vi "grab image.vi"(8 "error in (no error)":errorcluster, 10 "Image In":T1, 11 "Camera":T2) -> (0 "error out":errorcluster, 2 "Image Out":T1, 3 "Camera out":T2)   [LabVIEW 2022 SP3, in "Vision.lvlib"]
uses:
  Vision.lvlib
  camera.ctl
  camera driver.ctl
  <vilib>/vision/Image Controls.llb/IMAQ Image.ctl
  <vilib>/userDefined/High Color/IMAQdx.ctl
  C:/Users/Caleb/Desktop/nebraska-silicon-lab/pixel-gantry-control/Gantry/Shared Components/bin/uEyeDotNet.dll
  bin/uEyeDotNet.dll
  <vilib>/vision/driver/NI_Vision_Acquisition_Software.lvlib
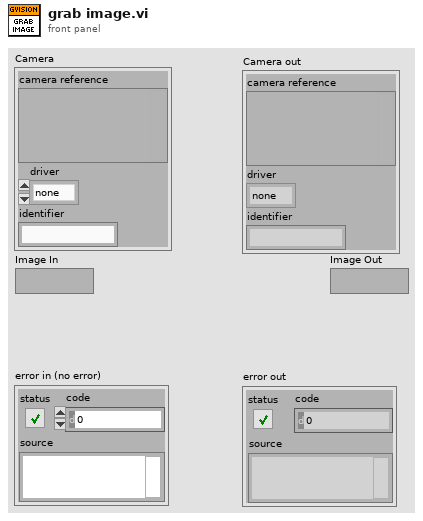
[diagram p1: front panel]
types:
  T1 = typedef "IMAQ Image.ctl" = refnum<image>
  T2 = typedef "Vision.lvlib/camera.ctl" = cluster{"camera reference":variant, "driver":T3, "identifier":string}
  T3 = typedef "Vision.lvlib/camera driver.ctl" = enum16{"none", "ueye", "wmf", "imaqdx"}
  T4 = typedef "IMAQdx.ctl" = refnum<k21>
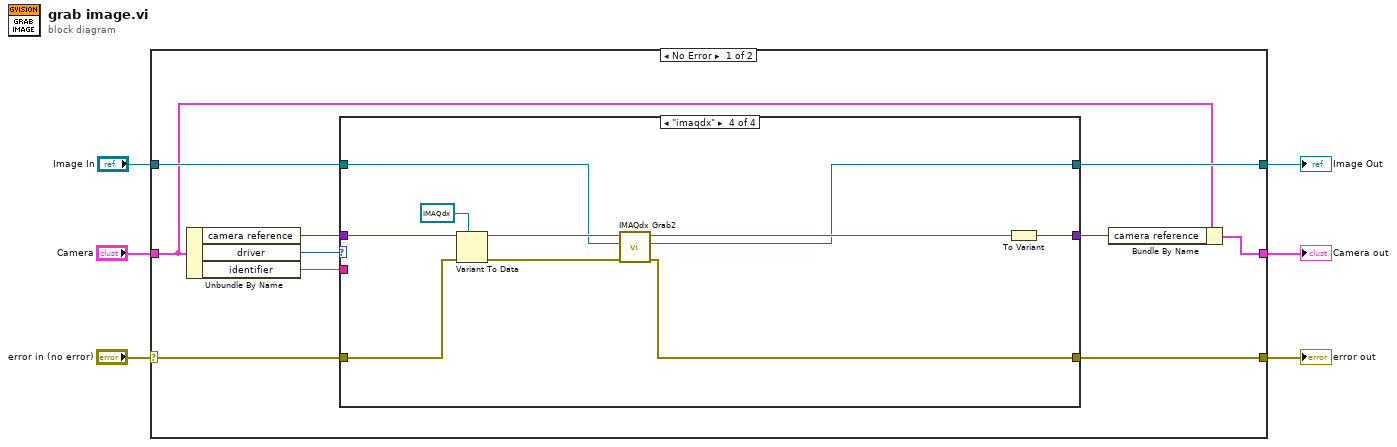
[diagram p0: block diagram]
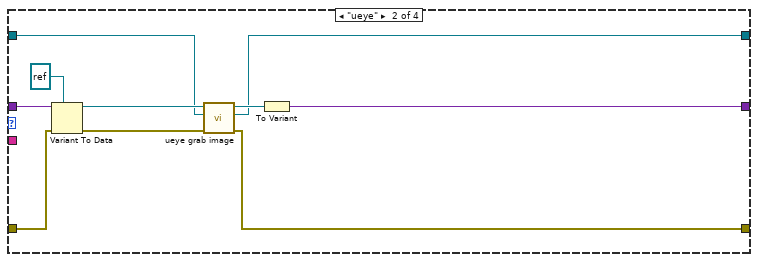
[diagram p3: hidden frame]
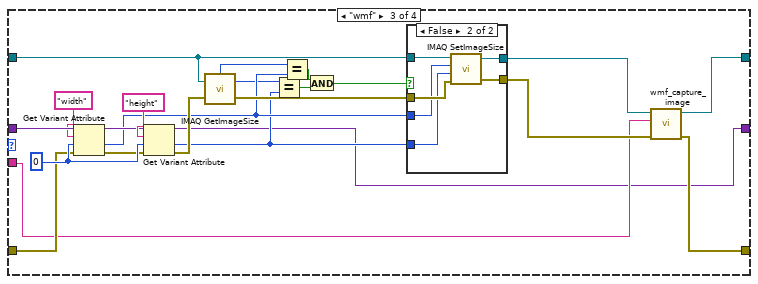
[diagram p4: hidden frame]
diagram:
  n1 = case shown="No Error" "error in (no error)" {
    selector: "error in (no error)" -> [w10 w72]
    tunnel: [w13 w72] -> w5
    tunnel: "Camera" -> [w9 w71]
    tunnel: [w8 w71] -> w3
    tunnel: [w12 _] -> w2
    tunnel: "Image In" -> [w11 _]
    frame No Error {
      n2 = Unbundle By Name(w9) -> ("camera reference"=w15:variant, "driver"=w16:T3, "identifier"=w14:string)
      n3 = case shown="\"imaqdx\"" w16 {
        tunnel: w15 -> [w18 w29 w52 w70]
        tunnel: w14 -> [_ _ w41 _]
        tunnel: w10 -> [w19 w27 w46 w69]
        tunnel: [w19 w20 w42 w61] -> w13
        tunnel: w11 -> [w17 w23 w38 w66]
        tunnel: [w17 w21 w44 w62] -> w12
        tunnel: [w18 w26 w30 w63] -> w7
        frame "none" {
        }
        frame "ueye" {
          n4 = Variant To Data(error in=w27, type=refnum<k24> refnum ("reference"), Variant=w29) -> (data=w25:refnum<k24>, error out=w24:errorcluster)
          n5 = call "ueye grab image.vi"("error in (no error)"=w24, "Image In"=w23, "Camera in"=w25) -> ("error out"=w20:errorcluster, "Image Out"=w21:T1, "Camera out"=w22:refnum<k24>)  [unwired: 6 in]
          n6 = To Variant(anything=w22) -> (Variant=w26:variant)
        }
        frame "wmf" {
          w48 = 0
          n7 = Get Variant Attribute(Variant=w52, name="width", default value (empty Variant)=w48, error in=w46) -> (duplicate Variant=w49:variant, value=w34:i32, error out=w47:errorcluster)  [unwired: 1 out]
          n8 = Get Variant Attribute(Variant=w49, name="height", default value (empty Variant)=w48, error in=w47) -> (duplicate Variant=w30:variant, value=w32:i32, error out=w40:errorcluster)  [unwired: 1 out]
          n9 = call "IMAQ GetImageSize"("Image"=w38, "error in (no error)"=w40) -> ("Y Resolution"=w33:i32, "X Resolution"=w35:i32, "error out"=w39:errorcluster)  [unwired: 2 in]
          n10 = Equal?(x=w33, y=w32) -> (x = y?=w36:bool)
          n11 = Equal?(x=w35, y=w34) -> (x = y?=w37:bool)
          n12 = And(x=w37, y=w36) -> (x .and. y?=w31:bool)
          n13 = case shown="False" w31 {
            tunnel: [w54 w60] -> w45
            tunnel: [w53 w59] -> w43
            tunnel: w39 -> [w53 w58]
            tunnel: w38 -> [w54 w57]
            tunnel: w34 -> [_ w56]
            tunnel: w32 -> [_ w55]
            frame True {
            }
            frame False {
              n14 = call "IMAQ SetImageSize"("error in (no error)"=w58, "Y Resolution"=w55, "X Resolution"=w56, "Image"=w57) -> ("error out"=w59:errorcluster, "Image Out"=w60:T1)  [unwired: 1 in]
            }
          }
          n15 = call "wmf_capture_image.vi"("error in (no error)"=w43, "identifier"=w41, "Image in"=w45) -> ("error out"=w42:errorcluster, "Image out"=w44:T1)  [unwired: 7 in]
        }
        frame "imaqdx" {
          n16 = Variant To Data(error in=w69, type=T4 refnum ("Session In"), Variant=w70) -> (data=w67:T4, error out=w65:errorcluster)
          n17 = call <vilib>:"IMAQdx Grab2.vi"("error in"=w65, "Image In"=w66, "Session In"=w67) -> ("error out"=w61:errorcluster, "Image Out"=w62:T1, "Session Out"=w64:T4)  [unwired: 5 in, 1 out]
          n18 = To Variant(anything=w64) -> (Variant=w63:variant)
        }
      }
      n19 = Bundle By Name(cluster=w9, "camera reference"=w7) -> (w8:T2)
    }
    frame Error {
    }
  }
  "error out" <- w5
  "Camera out" <- w3
  "Image Out" <- w2
